vi "CRYGet Graph Plot Info.vi"(10 "Plot Count":i32, 11 "Graph VI Ref":refnum<vi>) -> (2 "Flattened Plot Property":string, 3 "Flattened Scale Property":string)   [LabVIEW 2013]
uses:
  Control/CRYGraph Scale.ctl
panel:
  in  "Plot Setting":T1
  in  "Graph Info":T2={"X Scale.Maximum"=0.0, "X Scale.Minimum"=0.0, "Y0 Scale.Maximum"=0.0, "Y0 Scale.Minimum"=0.0, "Y1 Scale.Maximum"=0.0, "Y1 Scale.Minimum"=0.0, "X Scale.MapMode"=2, "Y1 Scale.MapMode"=2, "Y0 Scale.MapMode"=2, "ScaleFitX"=FALSE, "ScaleFitY"=FALSE, "ScaleFitY 2"=FALSE}
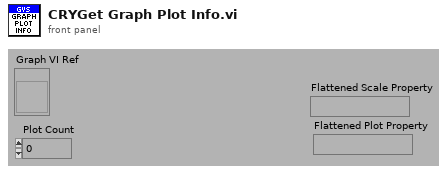
[diagram p1: front panel]
types:
  T1 = cluster{"Color":u32, "Interpolation":u8, "Point Style":u8, "Line Style":u8, "Point Color":u32, "Line Width":u8, "Bar Plot Style":u8, "Fill To":i16}
  T2 = typedef "CRYGraph Scale.ctl" = cluster{"X Scale.Maximum":dbl, "X Scale.Minimum":dbl, "Y0 Scale.Maximum":dbl, "Y0 Scale.Minimum":dbl, "Y1 Scale.Maximum":dbl, "Y1 Scale.Minimum":dbl, "X Scale.MapMode":u8, "Y1 Scale.MapMode":u8, "Y0 Scale.MapMode":u8, "ScaleFitX":bool, "ScaleFitY":bool, "ScaleFitY 2":bool}
  T3 = cluster{"Color":u32, "Interpolation":u8, "Point Style":u8, "Line Style":u8, "Point Color":u32, "Line Width":u8, "Bar Plot Style":u8, "Fill To":i16}[]
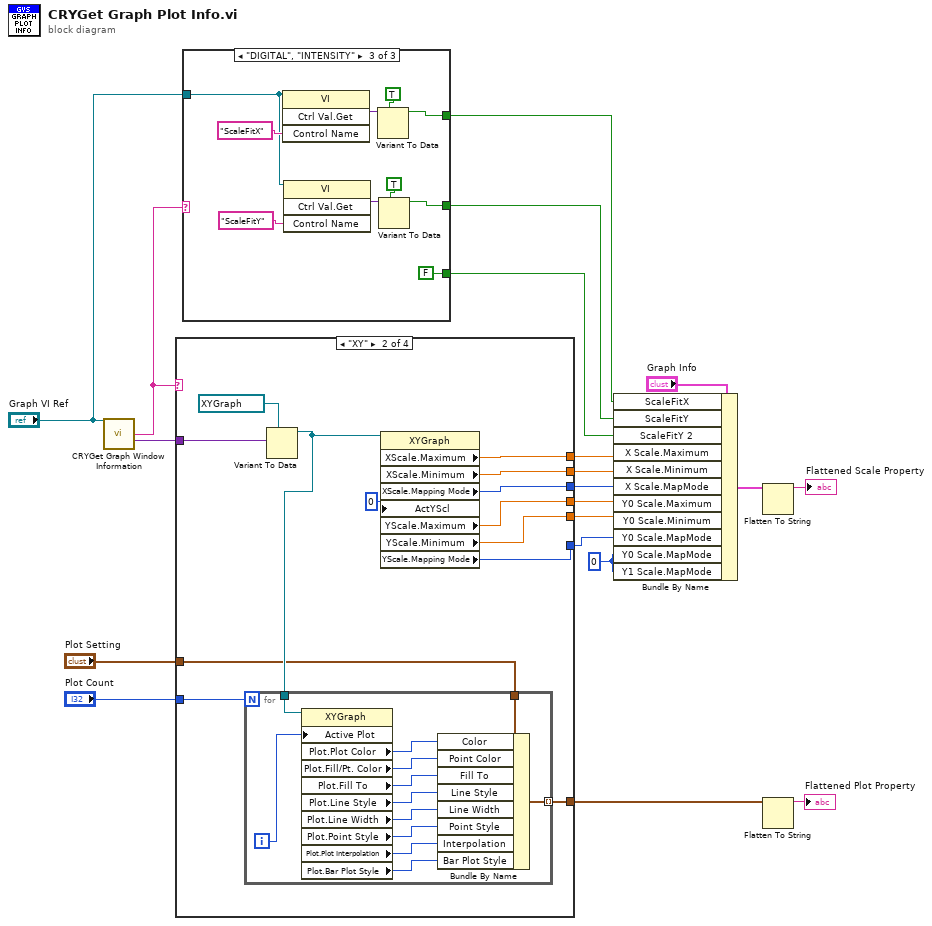
[diagram p0: block diagram]
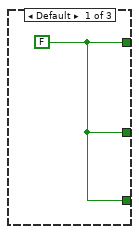
[diagram p2: hidden frame]
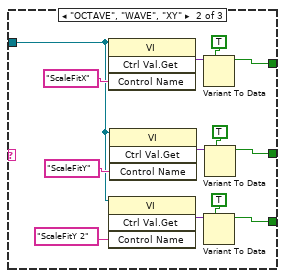
[diagram p3: hidden frame]
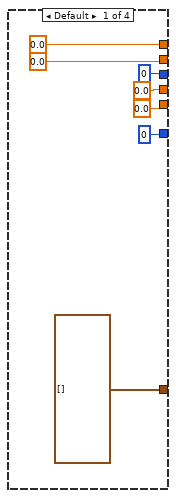
[diagram p4: hidden frame]
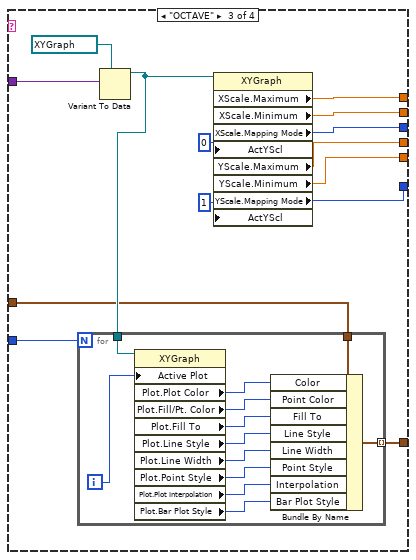
[diagram p5: hidden frame]
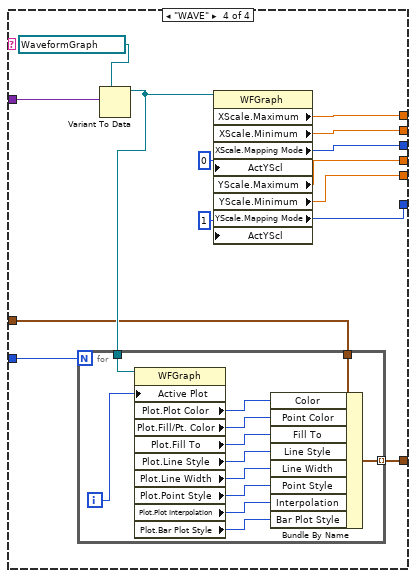
[diagram p6: hidden frame]
diagram:
  w13 = u8 0 ("Y1 Scale.Scale Fit")
  n1 = call "CRYGet Graph Window Information.vi"("pGraph VI In"="Graph VI Ref") -> ("Graph Type Out"=w5:string, "Graph Control Ref Out"=w12:variant)  [unwired: 4 in, 9 out]
  n2 = case shown="\"XY\"" w5 {
    tunnel: w12 -> [_ w40 w66 w92]
    tunnel: [0.0 ("XScale.Maximum") w38 w64 w91] -> w20
    tunnel: [0.0 ("XScale.Minimum") w37 w63 w90] -> w19
    tunnel: [0.0 ("YScale.Maximum") w30 w56 w83] -> w18
    tunnel: [0.0 ("YScale.Minimum") w35 w61 w88] -> w17
    tunnel: "Plot Count" -> [_ w33 w59 w86]
    tunnel: [T3 [] w32 w58 w85] -> w9
    tunnel: "Plot Setting" -> [_ w31 w57 w84]
    tunnel: [u8 0 ("XScale.Mapping Mode") w29 w54 w81] -> w15
    tunnel: [u8 0 ("YScale.Mapping Mode") w28 w53 w80] -> w14
    frame Default {
    }
    frame "XY" {
      n3 = Variant To Data(type=refnum<vi> refnum ("XY Graph"), Variant=w40) -> (data=w34:refnum<vi>)  [unwired: 1 in, 1 out]
      n4 = for {
        N: w33 -> [_]
        tunnel: w34 -> [w52]
        tunnel: w31 -> [w50]
        tunnel: [w42] -> w32 mode=indexing
        i -> [w51]
        n5 = property class="XYGraph"(reference=w52, "Active Plot"=w51) -> ("Plot.Plot Color"=w49:u32, "Plot.Fill/Pt. Color"=w48:u32, "Plot.Fill To"=w47:i16, "Plot.Line Style"=w46:u8, "Plot.Line Width"=w45:u8, "Plot.Point Style"=w44:u8, "Plot.Plot Interpolation"=w43:u8, "Plot.Bar Plot Style"=w41:u8)  [unwired: 1 in, 2 out]
        n6 = Bundle By Name(cluster=w50, "Color"=w49, "Point Color"=w48, "Fill To"=w47, "Line Style"=w46, "Line Width"=w45, "Point Style"=w44, "Interpolation"=w43, "Bar Plot Style"=w41) -> (w42:T1)
      }
      n7 = property class="XYGraph"(reference=w34, "ActYScl"=0 ("Active Y Scale")) -> ("XScale.Maximum"=w38:dbl, "XScale.Minimum"=w37:dbl, "XScale.Mapping Mode"=w29:u8, "YScale.Maximum"=w30:dbl, "YScale.Minimum"=w35:dbl, "YScale.Mapping Mode"=w28:u8)  [unwired: 1 in, 2 out]
    }
    frame "OCTAVE" {
      n8 = Variant To Data(type=refnum<vi> refnum ("XY Graph"), Variant=w66) -> (data=w60:refnum<vi>)  [unwired: 1 in, 1 out]
      n9 = for {
        N: w59 -> [_]
        tunnel: w60 -> [w78]
        tunnel: w57 -> [w76]
        tunnel: [w68] -> w58 mode=indexing
        i -> [w77]
        n10 = property class="XYGraph"(reference=w78, "Active Plot"=w77) -> ("Plot.Plot Color"=w75:u32, "Plot.Fill/Pt. Color"=w74:u32, "Plot.Fill To"=w73:i16, "Plot.Line Style"=w72:u8, "Plot.Line Width"=w71:u8, "Plot.Point Style"=w70:u8, "Plot.Plot Interpolation"=w69:u8, "Plot.Bar Plot Style"=w67:u8)  [unwired: 1 in, 2 out]
        n11 = Bundle By Name(cluster=w76, "Color"=w75, "Point Color"=w74, "Fill To"=w73, "Line Style"=w72, "Line Width"=w71, "Point Style"=w70, "Interpolation"=w69, "Bar Plot Style"=w67) -> (w68:T1)
      }
      n12 = property class="XYGraph"(reference=w60, "ActYScl"=0 ("Active Y Scale"), "ActYScl"=1 ("Active Y Scale")) -> ("XScale.Maximum"=w64:dbl, "XScale.Minimum"=w63:dbl, "XScale.Mapping Mode"=w54:u8, "YScale.Maximum"=w56:dbl, "YScale.Minimum"=w61:dbl, "YScale.Mapping Mode"=w53:u8)  [unwired: 1 in, 2 out]
    }
    frame "WAVE" {
      n13 = Variant To Data(type=refnum<vi> refnum ("WaveGraph Ref"), Variant=w92) -> (data=w87:refnum<vi>)  [unwired: 1 in, 1 out]
      n14 = for {
        N: w86 -> [_]
        tunnel: w87 -> [w104]
        tunnel: w84 -> [w102]
        tunnel: [w94] -> w85 mode=indexing
        i -> [w103]
        n15 = property class="WFGraph"(reference=w104, "Active Plot"=w103) -> ("Plot.Plot Color"=w101:u32, "Plot.Fill/Pt. Color"=w100:u32, "Plot.Fill To"=w99:i16, "Plot.Line Style"=w98:u8, "Plot.Line Width"=w97:u8, "Plot.Point Style"=w96:u8, "Plot.Plot Interpolation"=w95:u8, "Plot.Bar Plot Style"=w93:u8)  [unwired: 1 in, 2 out]
        n16 = Bundle By Name(cluster=w102, "Color"=w101, "Point Color"=w100, "Fill To"=w99, "Line Style"=w98, "Line Width"=w97, "Point Style"=w96, "Interpolation"=w95, "Bar Plot Style"=w93) -> (w94:T1)
      }
      n17 = property class="WFGraph"(reference=w87, "ActYScl"=0 ("Active Y Scale"), "ActYScl"=1 ("Active Y Scale")) -> ("XScale.Maximum"=w91:dbl, "XScale.Minimum"=w90:dbl, "XScale.Mapping Mode"=w81:u8, "YScale.Maximum"=w83:dbl, "YScale.Minimum"=w88:dbl, "YScale.Mapping Mode"=w80:u8)  [unwired: 1 in, 2 out]
    }
  }
  n18 = case shown="\"DIGITAL\", \"INTENSITY\"" w5 {
    tunnel: "Graph VI Ref" -> [_ w109 w122]
    tunnel: [w105 w108 w121] -> w3
    tunnel: [w105 w107 w120] -> w2
    tunnel: [w105 w106 FALSE] -> w1
    frame Default {
      w105 = FALSE
    }
    frame "OCTAVE", "WAVE", "XY" {
      n19 = invoke class="VI" method="Ctrl Val.Get"(reference=w109, "Control Name"="ScaleFitX") -> ("Get Control Value Variant"=w117:variant)  [unwired: 2 in, 3 out]
      n20 = invoke class="VI" method="Ctrl Val.Get"(reference=w109, "Control Name"="ScaleFitY 2") -> ("Get Control Value Variant"=w111:variant)  [unwired: 2 in, 3 out]
      n21 = invoke class="VI" method="Ctrl Val.Get"(reference=w109, "Control Name"="ScaleFitY") -> ("Get Control Value Variant"=w114:variant)  [unwired: 2 in, 3 out]
      n22 = Variant To Data(type=TRUE, Variant=w117) -> (data=w108:bool)  [unwired: 1 in, 1 out]
      n23 = Variant To Data(type=TRUE, Variant=w111) -> (data=w106:bool)  [unwired: 1 in, 1 out]
      n24 = Variant To Data(type=TRUE, Variant=w114) -> (data=w107:bool)  [unwired: 1 in, 1 out]
    }
    frame "DIGITAL", "INTENSITY" {
      n25 = invoke class="VI" method="Ctrl Val.Get"(reference=w122, "Control Name"="ScaleFitX") -> ("Get Control Value Variant"=w127:variant)  [unwired: 2 in, 3 out]
      n26 = invoke class="VI" method="Ctrl Val.Get"(reference=w122, "Control Name"="ScaleFitY") -> ("Get Control Value Variant"=w124:variant)  [unwired: 2 in, 3 out]
      n27 = Variant To Data(type=TRUE, Variant=w127) -> (data=w121:bool)  [unwired: 1 in, 1 out]
      n28 = Variant To Data(type=TRUE, Variant=w124) -> (data=w120:bool)  [unwired: 1 in, 1 out]
    }
  }
  n29 = Bundle By Name(cluster="Graph Info", "ScaleFitX"=w3, "ScaleFitY"=w2, "ScaleFitY 2"=w1, "X Scale.Maximum"=w20, "X Scale.Minimum"=w19, "X Scale.MapMode"=w15, "Y0 Scale.Maximum"=w18, "Y0 Scale.Minimum"=w17, "Y0 Scale.MapMode"=w14, "Y0 Scale.MapMode"=w13, "Y1 Scale.MapMode"=w13) -> (w11:T2)
  n30 = Flatten To String(anything=w11) -> (data string=→"Flattened Scale Property":string)  [unwired: 3 in, 2 out]
  n31 = Flatten To String(anything=w9) -> (data string=→"Flattened Plot Property":string)  [unwired: 3 in, 2 out]
